vi "FunctDataMgr.Default Tasks.vi"(8 "error in (no error)":errorcluster, 9 "Data In":variant, 10 "Task In":string, 11 "FunctDataMgr in":refnum<class "FunctDataMgr.lvclass">) -> (0 "error out":errorcluster, 2 "Not Fwd Data":bool, 3 "FunctDataMgr out":refnum<class "FunctDataMgr.lvclass">)   [LabVIEW 2024, in "FunctDataMgr.lvclass"]
uses:
  FunctDataMgr.lvclass
  Results/Result.Attribute.ctl
  Results/Result.Measurement and Attribute Item Status.ctl
  TestExec/TestExec.Local Result Data.ctl
  Results/Result.Numeric.ctl
  Results/Result.Limit Type.ctl
  Results/Result XML/TestResult.SW Item.ctl
  Reports/Report.Result FileDataObject.ctl
  Results/Result.Measurement Item.ctl
  FunctDataMgr.lvclass/FunctDataMgr.ctl
  <vilib>/KATE/SeqMgr/SeqMgr.Result Info.ctl
  <vilib>/KATE/SeqMgr/SeqMgr.Result State Enum.ctl
  Errors/Error.Error Code List.ctl
  <vilib>/KATE/SeqMgr/SeqMgr.lvlib
  Errors.lvlib
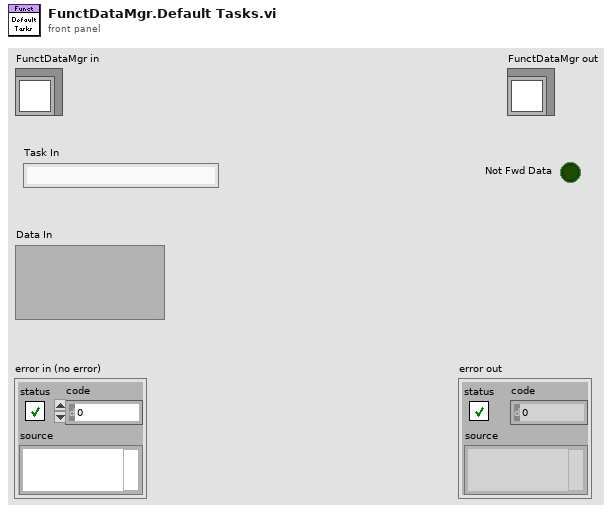
[diagram p1: front panel]
types:
  T1 = typedef "TestExec.Local Result Data.ctl" = cluster{"Attr":T2[], "Num":T4[], "UUT Props":string[][], "Vars":string[][], "SW Items":T6[], "Error":errorcluster, "Step":i32, "FileObjs":T7[], "MeasData":T8[]}
  T2 = typedef "Result.Attribute.ctl" = cluster{"Cnt":i32, "Step":string, "Category":string, "Name":string, "Value":string, "Status":T3, "Code":i32, "Desc":string, "Time":timestamp}
  T3 = typedef "Result.Measurement and Attribute Item Status.ctl" = i32
  T4 = typedef "Result.Numeric.ctl" = cluster{"Cnt":i32, "Step":string, "Category":string, "Name":string, "Value":dbl, "Units":string, "LimType":T5, "LL":dbl, "UL":dbl, "Status":T3, "Code":i32, "Desc":string, "Time":timestamp}
  T5 = typedef "Result.Limit Type.ctl" = enum16{"None", "EQ", "NE", "GT", "LT", "GE", "LE", "GTLT", "GELE", "GELT", "GTLE", "LTGT", "LEGE", "LEGT", "LTGE", "Contains", "NotContains"}
  T6 = typedef "TestResult.SW Item.ctl" = cluster{"Name":string, "PN":string, "Version":string, "Note":string}
  T7 = typedef "Report.Result FileDataObject.ctl" = cluster{"Cnt":i32, "Step":string, "Category":string, "Name":string, "Type":string, "File Name":string, "Time":string, "Path":path}
  T8 = typedef "Result.Measurement Item.ctl" = cluster{"Cnt":i32, "Step":string, "Category":string, "Name":string, "Value":string, "Units":string, "LimType":string, "LL":string, "UL":string, "Status":T3, "Code":i32, "Desc":string, "Time":timestamp}
  T9 = typedef "KATE_Lib.lvlib/SeqMgr.lvlib/SeqMgr.Result Info.ctl" = cluster{"State":T10, "Code":i32, "Description":string}
  T10 = typedef "KATE_Lib.lvlib/SeqMgr.lvlib/SeqMgr.Result State Enum.ctl" = enum16{"None", "Passing", "Failing", "PASS", "FAIL", "ABORT", "ERROR"}
  T11 = typedef "EQMF.lvlib/Errors.lvlib/Error.Error Code List.ctl" = i32
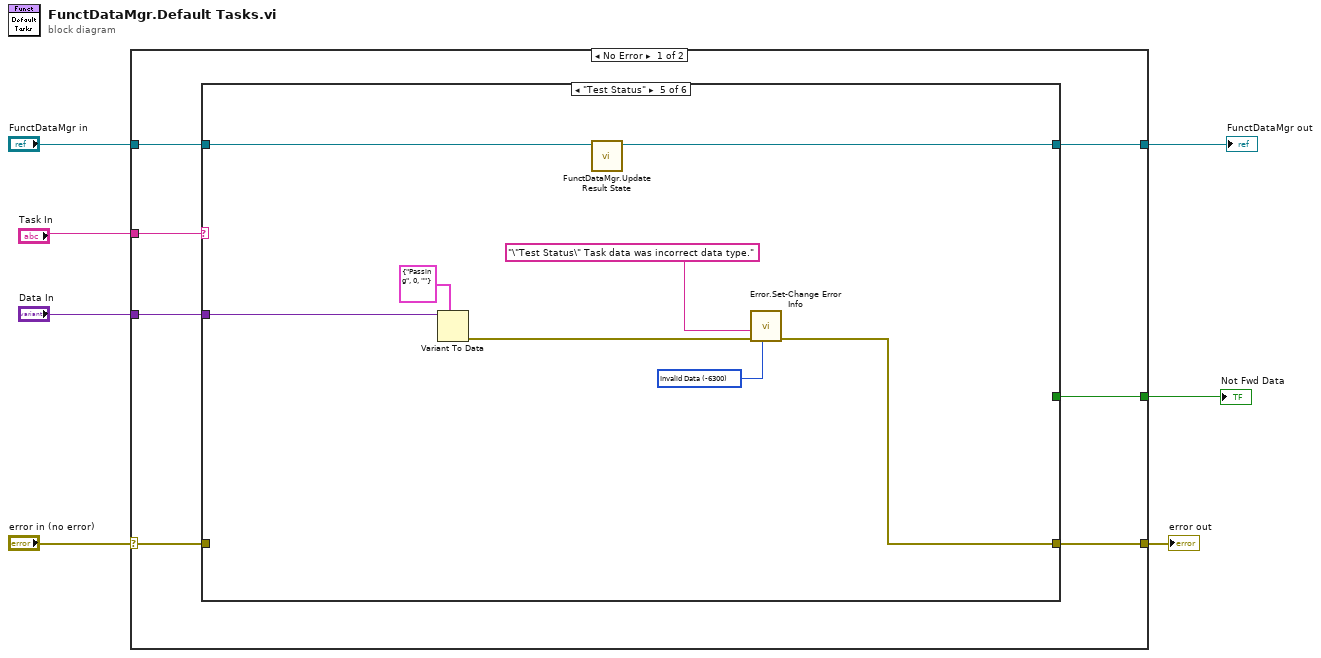
[diagram p0: block diagram]
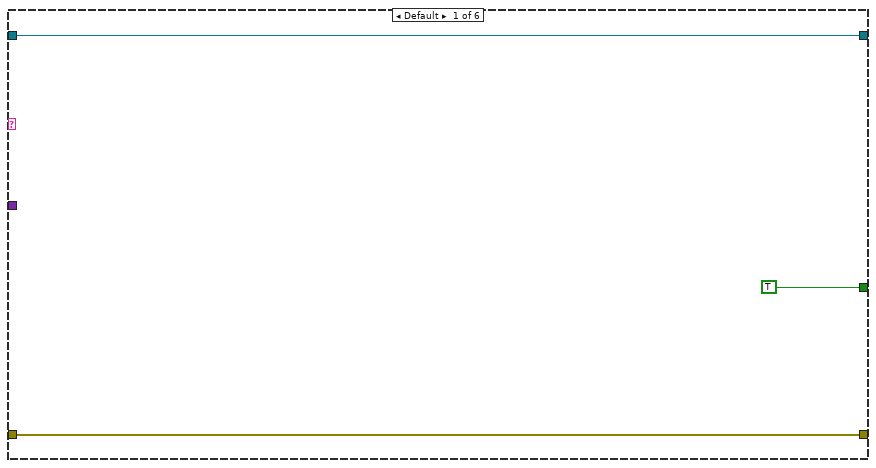
[diagram p2: hidden frame]
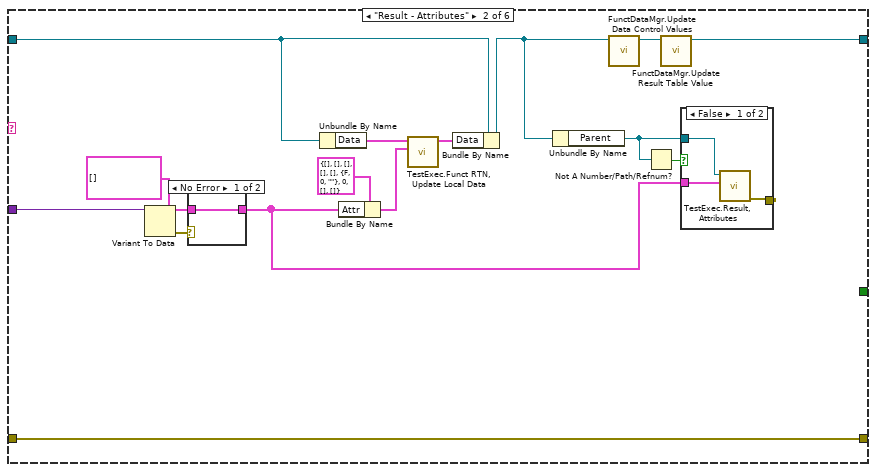
[diagram p3: hidden frame]
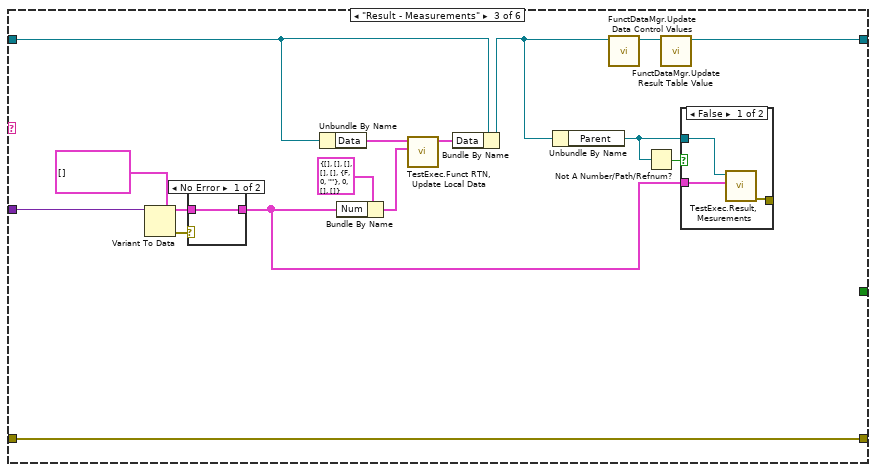
[diagram p6: hidden frame]
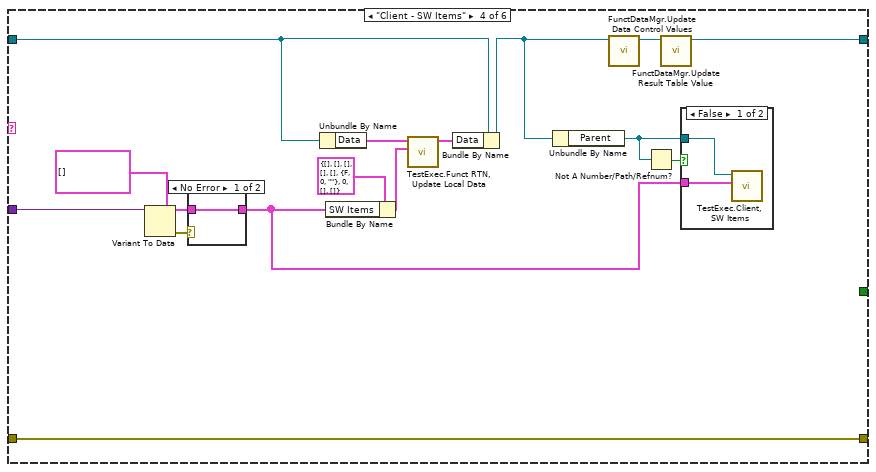
[diagram p9: hidden frame]
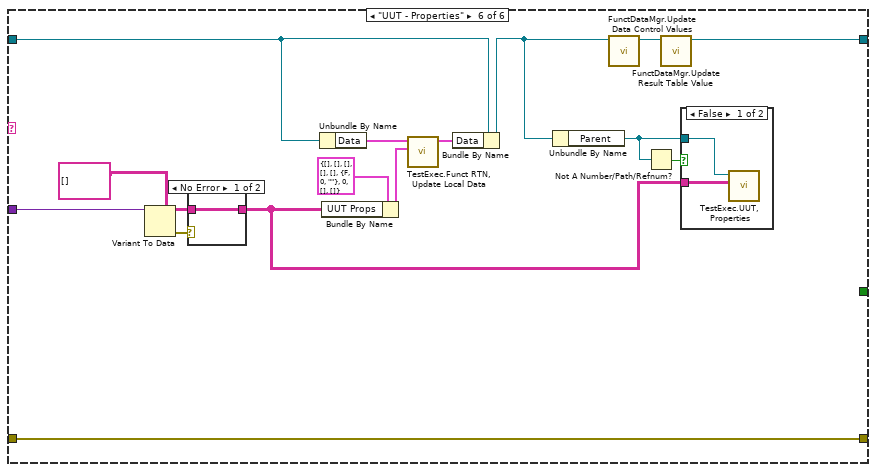
[diagram p12: hidden frame]
diagram:
  n1 = case shown="No Error" "error in (no error)" {
    selector: "error in (no error)" -> [w12 w105]
    tunnel: [w11 w105] -> w6
    tunnel: [w13 w104] -> w4
    tunnel: "FunctDataMgr in" -> [w14 w104]
    tunnel: "Task In" -> [w10 _]
    tunnel: "Data In" -> [w9 _]
    tunnel: [w8 _] -> w1
    frame No Error {
      n2 = case shown="\"Test Status\"" w10 {
        tunnel: w14 -> [w17 w32 w52 w72 w84 w99]
        tunnel: [w17 w31 w51 w71 w83 w98] -> w13
        tunnel: w12 -> [w15 w33 w53 w73 _ w100]
        tunnel: [w15 w33 w53 w73 w79 w100] -> w11
        tunnel: w9 -> [_ w30 w50 w70 w81 w97]
        tunnel: [TRUE _ _ _ _ _] -> w8
        frame Default {
        }
        frame "Result - Attributes" {
          n3 = Variant To Data(type=T2[] [] ("RTN Data.Attr"), Variant=w30) -> (data=w27:T2[], error out=w26:errorcluster)  [unwired: 1 in]
          n4 = case shown="No Error" w26 {
            tunnel: w27 -> [w37 _]
            tunnel: [w37 _] -> w18
            frame No Error {
            }
            frame Error {
            }
          }
          n5 = Unbundle By Name(w32) -> ("Data"=w29:T1)
          n6 = Bundle By Name(cluster=T1 {"Attr"=[], "Num"=[], "UUT Props"=[], "Vars"=[], "SW Items"=[], "Error"={"status"=FALSE, "code"=0, "source"=""}, "Step"=0, "FileObjs"=[], "MeasData"=[]} ("RTN Data"), "Attr"=w18) -> (w23:T1)
          n7 = call "TestExec.Funct RTN, Update Local Data.vi"("RTN Data"=w23, "Local Data"=w29) -> ("Local Data Out"=w28:T1)  [unwired: 9 in]
          n8 = Bundle By Name(cluster=w32, "Data"=w28) -> (w19:refnum<class "FunctDataMgr.lvclass">)
          n9 = Unbundle By Name(w19) -> ("Parent"=w21:refnum<queue>)
          n10 = call "FunctDataMgr.Update Data Control Values.vi"("FunctDataMgr in"=w19) -> ("FunctDataMgr out"=w22:refnum<class "FunctDataMgr.lvclass">)  [unwired: 9 in, 1 out]
          n11 = Not A Number/Path/Refnum?(number/path/refnum=w21) -> (NaN/Path/Refnum?=w20:bool)
          n12 = call "FunctDataMgr.Update Result Table Value.vi"("FunctDataMgr in"=w22) -> ("FunctDataMgr out"=w31:refnum<class "FunctDataMgr.lvclass">)  [unwired: 9 in, 1 out]
          n13 = case shown="False" w20 {
            tunnel: w18 -> [w36 _]
            tunnel: [w35 _] -> _
            tunnel: w21 -> [w34 _]
            frame False {
              n14 = call "TestExec.Result, Attributes.vi"("Attributes"=w36, "Q In"=w34) -> ("error out"=w35:errorcluster)  [unwired: 9 in]
            }
            frame True {
            }
          }
        }
        frame "Result - Measurements" {
          n15 = Variant To Data(type=T4[] [] ("RTN Data.Num"), Variant=w50) -> (data=w47:T4[], error out=w46:errorcluster)  [unwired: 1 in]
          n16 = case shown="No Error" w46 {
            tunnel: w47 -> [w57 _]
            tunnel: [w57 _] -> w39
            frame No Error {
            }
            frame Error {
            }
          }
          n17 = Unbundle By Name(w52) -> ("Data"=w49:T1)
          n18 = Bundle By Name(cluster=T1 {"Attr"=[], "Num"=[], "UUT Props"=[], "Vars"=[], "SW Items"=[], "Error"={"status"=FALSE, "code"=0, "source"=""}, "Step"=0, "FileObjs"=[], "MeasData"=[]} ("RTN Data"), "Num"=w39) -> (w44:T1)
          n19 = call "TestExec.Funct RTN, Update Local Data.vi"("RTN Data"=w44, "Local Data"=w49) -> ("Local Data Out"=w48:T1)  [unwired: 9 in]
          n20 = Bundle By Name(cluster=w52, "Data"=w48) -> (w40:refnum<class "FunctDataMgr.lvclass">)
          n21 = Unbundle By Name(w40) -> ("Parent"=w42:refnum<queue>)
          n22 = call "FunctDataMgr.Update Data Control Values.vi"("FunctDataMgr in"=w40) -> ("FunctDataMgr out"=w43:refnum<class "FunctDataMgr.lvclass">)  [unwired: 9 in, 1 out]
          n23 = Not A Number/Path/Refnum?(number/path/refnum=w42) -> (NaN/Path/Refnum?=w41:bool)
          n24 = call "FunctDataMgr.Update Result Table Value.vi"("FunctDataMgr in"=w43) -> ("FunctDataMgr out"=w51:refnum<class "FunctDataMgr.lvclass">)  [unwired: 9 in, 1 out]
          n25 = case shown="False" w41 {
            tunnel: w39 -> [w54 _]
            tunnel: [w55 _] -> _
            tunnel: w42 -> [w56 _]
            frame False {
              n26 = call "TestExec.Result, Mesurements.vi"("Numeric"=w54, "Q In"=w56) -> ("error out"=w55:errorcluster)  [unwired: 9 in]
            }
            frame True {
            }
          }
        }
        frame "Client - SW Items" {
          n27 = Variant To Data(type=T6[] [] ("RTN Data.Num"), Variant=w70) -> (data=w67:T6[], error out=w66:errorcluster)  [unwired: 1 in]
          n28 = case shown="No Error" w66 {
            tunnel: w67 -> [w76 _]
            tunnel: [w76 _] -> w59
            frame No Error {
            }
            frame Error {
            }
          }
          n29 = Unbundle By Name(w72) -> ("Data"=w69:T1)
          n30 = Bundle By Name(cluster=T1 {"Attr"=[], "Num"=[], "UUT Props"=[], "Vars"=[], "SW Items"=[], "Error"={"status"=FALSE, "code"=0, "source"=""}, "Step"=0, "FileObjs"=[], "MeasData"=[]} ("RTN Data"), "SW Items"=w59) -> (w64:T1)
          n31 = call "TestExec.Funct RTN, Update Local Data.vi"("RTN Data"=w64, "Local Data"=w69) -> ("Local Data Out"=w68:T1)  [unwired: 9 in]
          n32 = Bundle By Name(cluster=w72, "Data"=w68) -> (w60:refnum<class "FunctDataMgr.lvclass">)
          n33 = Unbundle By Name(w60) -> ("Parent"=w62:refnum<queue>)
          n34 = call "FunctDataMgr.Update Data Control Values.vi"("FunctDataMgr in"=w60) -> ("FunctDataMgr out"=w63:refnum<class "FunctDataMgr.lvclass">)  [unwired: 9 in, 1 out]
          n35 = Not A Number/Path/Refnum?(number/path/refnum=w62) -> (NaN/Path/Refnum?=w61:bool)
          n36 = call "FunctDataMgr.Update Result Table Value.vi"("FunctDataMgr in"=w63) -> ("FunctDataMgr out"=w71:refnum<class "FunctDataMgr.lvclass">)  [unwired: 9 in, 1 out]
          n37 = case shown="False" w61 {
            tunnel: w59 -> [w74 _]
            tunnel: w62 -> [w75 _]
            frame False {
              n38 = call "TestExec.Client, SW Items.vi"("SW Items"=w74, "Q In"=w75) -> ()  [unwired: 8 in, 2 out]
            }
            frame True {
            }
          }
        }
        frame "Test Status" {
          w78 = T11 -6300 items=["No Error"=0, "Abort"=-2, "Misc"=-5000, "Fixture Error"=-5100, "File IO - General"=-5200, "FIle IO - Config Error"=-5201, "Instrument - General"=-5300, "Instrument - Serial Com"=-5301, "Instrument - Camera"=-5302, "Instrument - PS"=-5303, "Instrument - Oscilloscope"=-5304, "Instrument - Function Gen"=-5305, "Instrument - Load"=-5306, "Instrument - Meter"=-5307, "Instrument - Power Control"=-5308, "Instrument - Motion"=-5309, "Instrument - RF"=-5310, "System Exe"=-5400, "Image Processing"=-5500, "Communication"=-5600, "Script - Syntax Error"=-6000, "Script - Invalid Name or Param"=-6100, "Script - Timeout"=-6200, "Invalid Data"=-6300, "FW Update Error"=-6500] ("Std Code")
          n39 = Variant To Data(type=T9 {"State"=enum."Passing", "Code"=0, "Description"=""} ("ResultState"), Variant=w81) -> (error out=w80:errorcluster)  [unwired: 1 in, 1 out]
          n40 = call "FunctDataMgr.Update Result State.vi"("FunctDataMgr in"=w84) -> ("FunctDataMgr out"=w83:refnum<class "FunctDataMgr.lvclass">)  [unwired: 9 in, 1 out]
          n41 = call "Error.Set-Change Error Info.vi"("Std Code"=w78, "error in"=w80, "Description"="\"Test Status\" Task data was incorrect data type.") -> ("error out"=w79:errorcluster)  [unwired: 8 in]
        }
        frame "UUT - Properties" {
          n42 = Variant To Data(type=string[][] [] ("UUT Props"), Variant=w97) -> (data=w94:string[][], error out=w93:errorcluster)  [unwired: 1 in]
          n43 = case shown="No Error" w93 {
            tunnel: w94 -> [w103 _]
            tunnel: [w103 _] -> w86
            frame No Error {
            }
            frame Error {
            }
          }
          n44 = Unbundle By Name(w99) -> ("Data"=w96:T1)
          n45 = Bundle By Name(cluster=T1 {"Attr"=[], "Num"=[], "UUT Props"=[], "Vars"=[], "SW Items"=[], "Error"={"status"=FALSE, "code"=0, "source"=""}, "Step"=0, "FileObjs"=[], "MeasData"=[]} ("RTN Data"), "UUT Props"=w86) -> (w91:T1)
          n46 = call "TestExec.Funct RTN, Update Local Data.vi"("RTN Data"=w91, "Local Data"=w96) -> ("Local Data Out"=w95:T1)  [unwired: 9 in]
          n47 = Bundle By Name(cluster=w99, "Data"=w95) -> (w87:refnum<class "FunctDataMgr.lvclass">)
          n48 = Unbundle By Name(w87) -> ("Parent"=w89:refnum<queue>)
          n49 = call "FunctDataMgr.Update Data Control Values.vi"("FunctDataMgr in"=w87) -> ("FunctDataMgr out"=w90:refnum<class "FunctDataMgr.lvclass">)  [unwired: 9 in, 1 out]
          n50 = Not A Number/Path/Refnum?(number/path/refnum=w89) -> (NaN/Path/Refnum?=w88:bool)
          n51 = call "FunctDataMgr.Update Result Table Value.vi"("FunctDataMgr in"=w90) -> ("FunctDataMgr out"=w98:refnum<class "FunctDataMgr.lvclass">)  [unwired: 9 in, 1 out]
          n52 = case shown="False" w88 {
            tunnel: w86 -> [w101 _]
            tunnel: w89 -> [w102 _]
            frame False {
              n53 = call "TestExec.UUT, Properties.vi"("UUT Properties"=w101, "Q In"=w102) -> ()  [unwired: 9 in, 1 out]
            }
            frame True {
            }
          }
        }
      }
    }
    frame Error {
    }
  }
  "error out" <- w6
  "FunctDataMgr out" <- w4
  "Not Fwd Data" <- w1
